vi "GetCtrlsToUndo.vi"(8 "error in":errorcluster, 11 "References\nfor Controls\non parent":refnum<vi>[](array[refnum])) -> (0 "error out":errorcluster, 3 "Parent's Controls":refnum<vi>[](array[refnum]) caption="References\nfor Controls\non parent (excluded\nindicators, latch booleans,\ncluster containers, radio\nbuttons containers)", 4 "Index":i32[](array[numeric]), 6 "Initial Values":variant[](array[variant]))   [LabVIEW 2015, in "UndoLibrary.lvlib"]
doc: "This VI excludes the references for:\n- indicators\n- booleans with latch mechanical action, because their value can not be read nor written via property nodes"
uses:
  UndoLibrary.lvlib
panel:
  # "This VI excludes the references for:\n- indicators\n- booleans with latch mechanical action, because their value can not be read nor written via property nodes\n- clusters and radio buttons, because the elements inside of them are already being referenced separately"
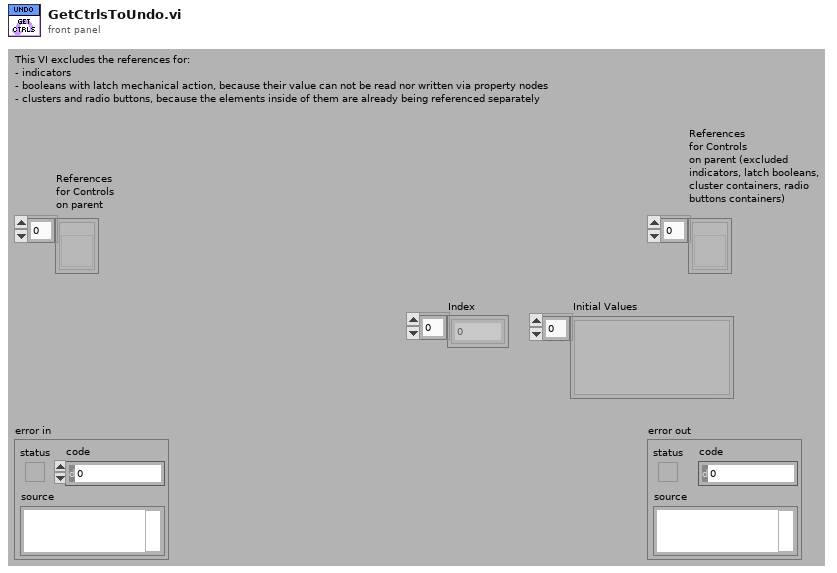
[diagram p1: front panel]
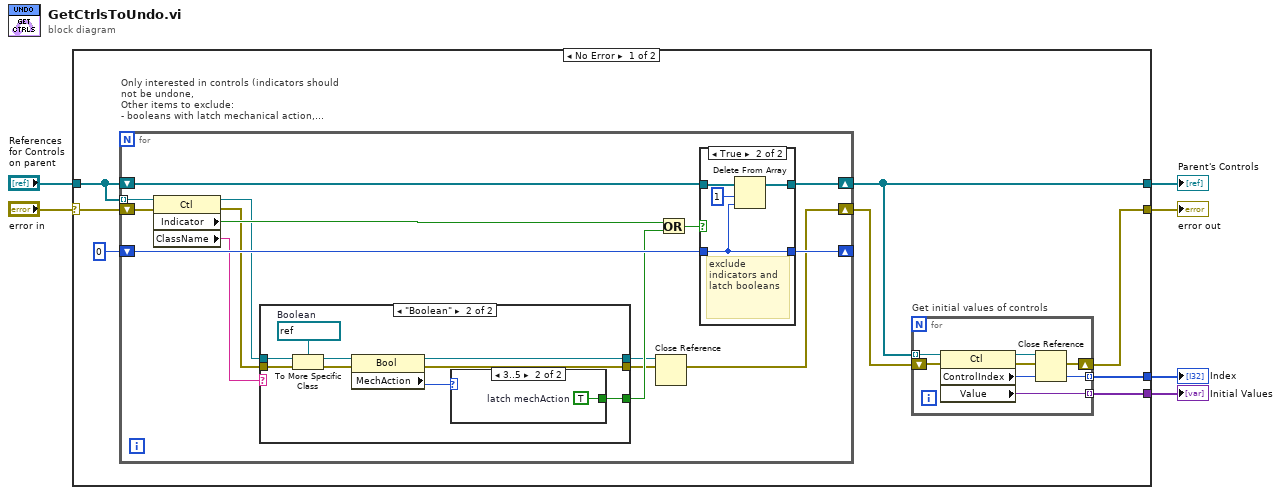
[diagram p0: block diagram]
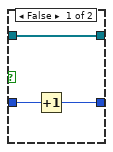
[diagram p4: hidden frame]
diagram:
  n1 = case shown="No Error" "error in" {
    selector: "error in" -> [w12 w55]
    tunnel: "References\nfor Controls\non parent" -> [w13 w54]
    tunnel: [w9 w55] -> w5
    tunnel: [w11 w54] -> w4
    tunnel: [w8 _] -> w1
    tunnel: [w7 _] -> w2
    frame No Error {
      n2 = for "Only interested in controls (indicators should not be undone,\nOther items to exclude:\n- booleans with latch mechanical action, because their value can not be read nor written via property nodes\n- clusters and radio buttons, because the elements inside of them are already being referenced separately" {
        tunnel: w13 -> [w34] mode=indexing
        shift-right: [w21] -> w10
        shift-left: w12 -> [w33]
        shift-right: [w30] -> w11
        shift-left: w13 -> [w31]
        shift-right: [w28] -> _
        shift-left: 0 -> [w29]
        n3 = property class="Ctl"(reference=w34, error in=w33) -> (reference out=w24:refnum<vi>, error out=w22:errorcluster, "Indicator"=w32:bool, "ClassName"=w27:string)
        n4 = case shown="\"Boolean\"" w27 {
          tunnel: w24 -> [w36 w45]
          tunnel: [_ w41] -> w25
          tunnel: [w36 w40] -> w23
          tunnel: w22 -> [w35 w39]
          tunnel: [w35 w37] -> w21
          frame "False", Default {
          }
          frame "Boolean" {
            w44 = refnum<vi> refnum  # Boolean
            n5 = To More Specific Class(target class=w44, reference=w45, error in=w39) -> (specific class reference=w43:refnum<vi>, error out=w38:errorcluster)
            n6 = property class="Bool"(reference=w43, error in=w38) -> (reference out=w40:refnum<vi>, error out=w37:errorcluster, "MechAction"=w42:u32)
            n7 = case shown="3..5" w42 {
              tunnel: [_ w46] -> w41
              frame Default {
              }
              frame 3..5 {
                w46 = TRUE  # latch mechAction
              }
            }
          }
        }
        n8 = Close Reference(reference=w23) -> ()  [unwired: 1 in, 1 out]
        n9 = Or(x=w32, y=w25) -> (x .or. y?=w26:bool)
        n10 = case shown="True" w26 {
          tunnel: w31 -> [w47 w53]
          tunnel: w29 -> [w49 w50]
          tunnel: [w48 w50] -> w28
          tunnel: [w47 w51] -> w30
          frame False {
            n11 = Increment(x=w49) -> (x+1=w48:i32)
          }
          frame True {
            # "exclude indicators and latch booleans"
            n12 = Delete From Array(array=w53, length=1, index=w50) -> (array with subset deleted=w51:refnum<vi>[])  [unwired: 1 out]
          }
        }
      }
      n13 = for "Get initial values of controls" {
        tunnel: w11 -> [w20] mode=indexing
        shift-right: [w18] -> w9
        shift-left: w10 -> [w19]
        tunnel: [w16] -> w8 mode=indexing
        tunnel: [w15] -> w7 mode=indexing
        n14 = property class="Ctl"(reference=w20, error in=w19) -> (reference out=w17:refnum<vi>, error out=w18:errorcluster, "ControlIndex"=w16:i32, "Value"=w15:variant)
        n15 = Close Reference(reference=w17) -> ()  [unwired: 1 in, 1 out]
      }
    }
    frame Error {
    }
  }
  "error out" <- w5
  "Parent's Controls" <- w4
  "Initial Values" <- w2
  "Index" <- w1
